vi "Add new user manually.vi"   [LabVIEW 2020, in "Data Manager.lvclass"]
uses:
  Data Manager.lvclass
  Application/Globals.vi
  Application/Application.lvlib
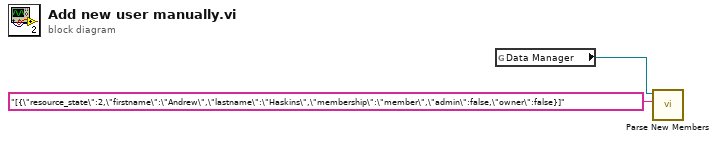
[diagram p0: block diagram]
diagram:
  n1 = global read "Globals.vi" "Data Manager"() -> (w2:refnum<class "Data Manager.lvclass">)
  n2 = call-dynamic "Parse New Members.vi"("Club Members JSON"="[{\"resource_state\":2,\"firstname\":\"Andrew\",\"lastname\":\"Haskins\",\"membership\":\"member\",\"admin\":false,\"owner\":false}]", "Data Manager in"=w2) -> ()  [unwired: 8 in, 2 out]
